vi "Modulator.vi"(8 "error in (no error)":errorcluster, 11 "ISO 14443 A DOWN in":refnum<class "ISO 14443 A DOWN.lvclass">) -> (0 "error out":errorcluster, 2 "Waveform out":waveform(dbl), 3 "ISO 14443 A DOWN out":refnum<class "ISO 14443 A DOWN.lvclass">)   [LabVIEW 2019, in "ISO 14443 A DOWN.lvclass"]
uses:
  ISO 14443 A DOWN.lvclass
  TypeDef/Store.ctl
  ISO 14443 A DOWN.lvclass/ISO 14443 A DOWN.ctl
  <vilib>/addons/Modulation/Analog/MT Modulate AM (DSB).vi
  <vilib>/addons/Modulation/Analog/MT Upconvert Baseband (Real).vi
  <vilib>/addons/Modulation/niAMT.lvlib
  RFID system.lvclass
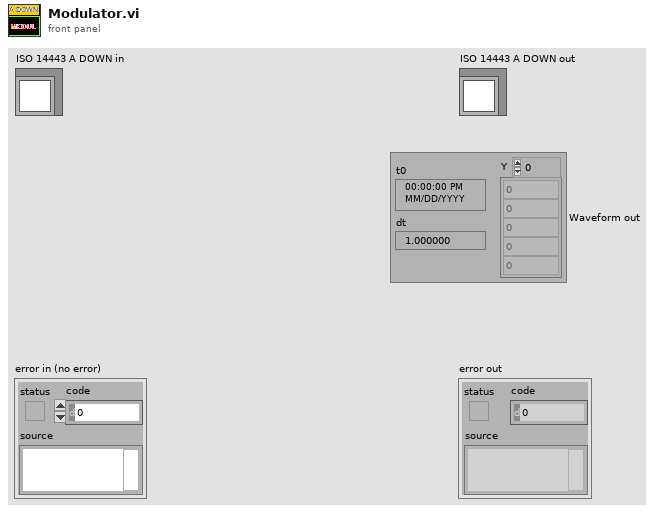
[diagram p1: front panel]
types:
  T1 = typedef "Store.ctl" = enum16{"envelope", "noise", "demSubCar", "CH_frame", "Decode", "demodulate", "in", "out", "sum", "subCarrier", "frame", "command", "encode", "modulate", "encode_UP", "modulate_up", "demod_up", "envelop_up", "sum_up", "out_up", "in_up"}
  T2 = typedef "niAMT.lvlib/Complex Data Waveform.ctl" = cluster{"t0":dbl, "dt":dbl, "Y":cdb[]}
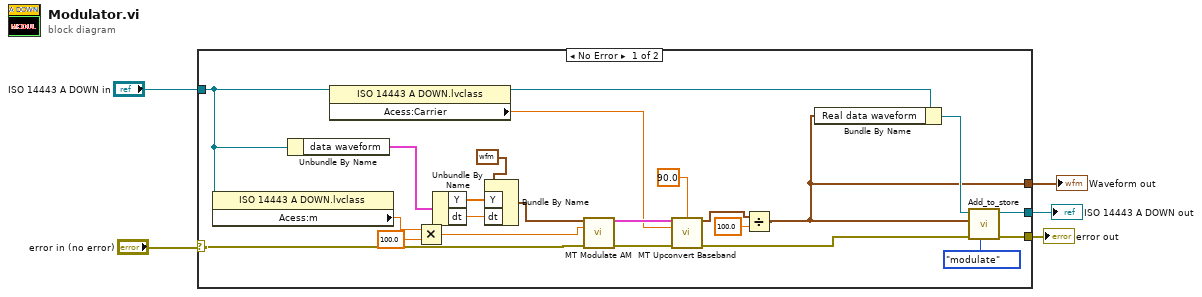
[diagram p0: block diagram]
diagram:
  n1 = case shown="No Error" "error in (no error)" {
    selector: "error in (no error)" -> [w20 w29]
    tunnel: [w16 w29] -> w4
    tunnel: "ISO 14443 A DOWN in" -> [w12 w30]
    tunnel: [w13 w30] -> w2
    tunnel: [w6 _] -> w1
    frame No Error {
      n2 = property class="ISO 14443 A DOWN.lvclass"(reference=w12) -> ("Acess:m"=w11:dbl)  [unwired: 1 in, 2 out]
      n3 = Unbundle By Name(w12) -> ("data waveform"=w21:T2)
      n4 = property class="ISO 14443 A DOWN.lvclass"(reference=w12) -> (reference out=w19:refnum<class "ISO 14443 A DOWN.lvclass">, "Acess:Carrier"=w18:dbl)  [unwired: 1 in, 1 out]
      n5 = Multiply(x=w11, y=100.0) -> (x*y=w9:dbl)
      n6 = Unbundle By Name(w21) -> ("Y"=w27:cdb[], "dt"=w28:dbl)
      n7 = Bundle By Name(cluster=waveform(cdb) {"t0"=timestamp(0 s since 1904-01-01), "dt"=1.0, "Y"=[]} ("waveform"), "Y"=w27, "dt"=w28) -> (w25:waveform(cdb))
      n8 = call-poly <vilib>:"MT Modulate AM.vi"("message signal"=w25, "modulation index"=w9, "error in (no error)"=w20) -> ("AM modulated waveform"=w26:cluster{"t0":dbl, "dt":dbl, "Y":cdb[]}, "error out"=w24:errorcluster)  [unwired: 11 in]
      n9 = call-poly <vilib>:"MT Upconvert Baseband.vi"("baseband waveform (complex)"=w26, "initial phase (deg)"=90.0, "carrier frequency (Hz)"=w18, "error in (no error)"=w24) -> ("passband waveform"=w8:waveform(dbl), "error out"=w17:errorcluster)  [unwired: 10 in]
      n10 = Divide(x=w8, y=100.0) -> (x/y=w6:waveform(dbl))
      n11 = Bundle By Name(cluster=w19, "Real data waveform"=w6) -> (w14:refnum<class "ISO 14443 A DOWN.lvclass">)
      n12 = call "Add_to_store.vi"("Store"=Store."modulate", "error in (no error)"=w17, "Waveform"=w6, "RFID system in"=w14) -> ("error out"=w16:errorcluster, "RFID system out"=w13:refnum<class "ISO 14443 A DOWN.lvclass">)  [unwired: 6 in]
    }
    frame Error {
    }
  }
  "error out" <- w4
  "ISO 14443 A DOWN out" <- w2
  "Waveform out" <- w1
